vi "Fix_multi_header_bug.vi"(1 "Raw data File to Read":path) -> (0 "Raw data File to Read Out":path)   [LabVIEW 2010]
uses:
  Globals/Meas_global.vi
  Globals/Constants_global.vi
panel:
  out "character string":string
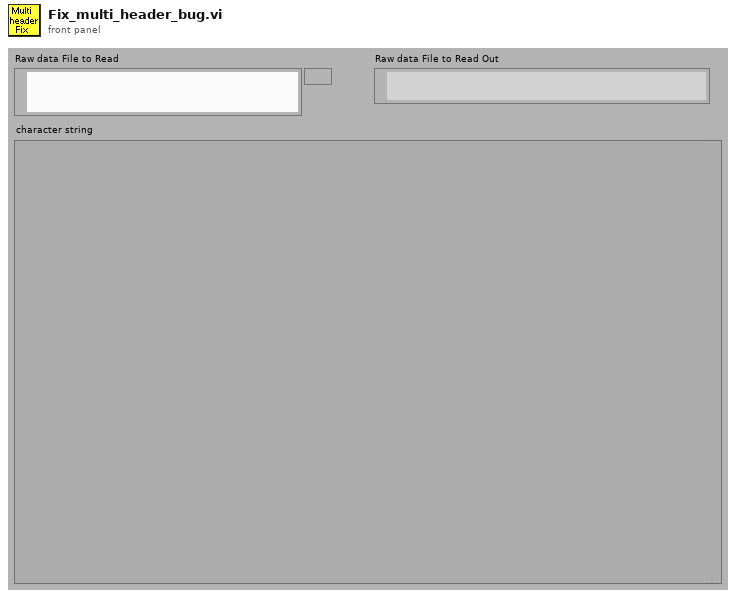
[diagram p1: front panel]
types:
  T1 = enum16{"read/write", "read-only", "write-only", "write-only (truncate)"}
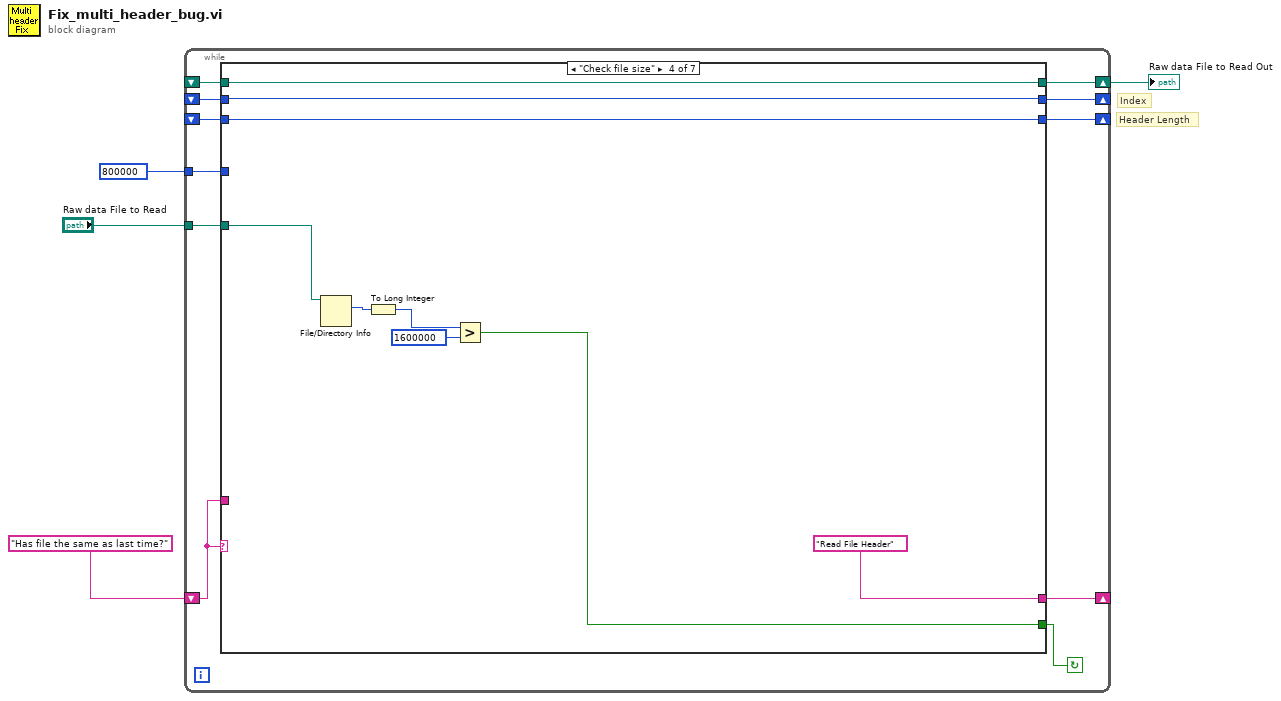
[diagram p0: block diagram]
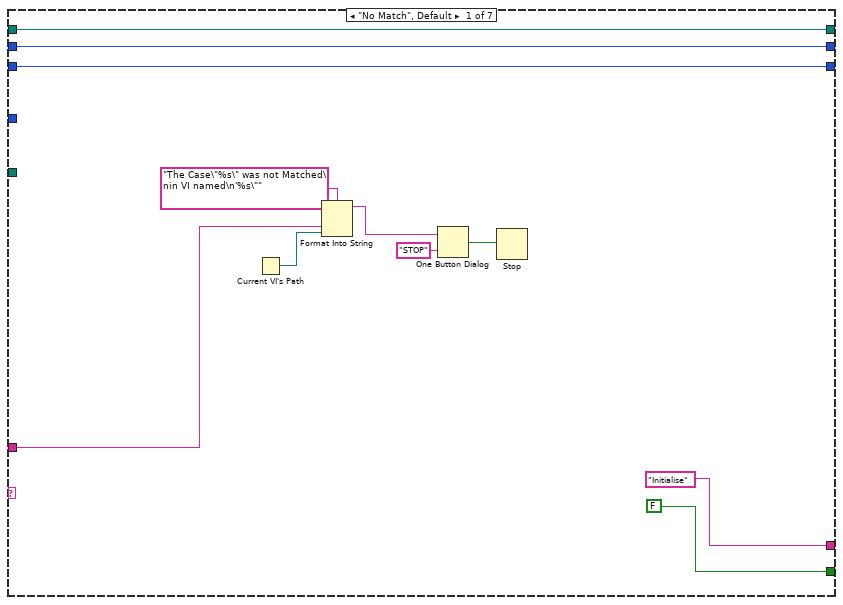
[diagram p2: hidden frame]
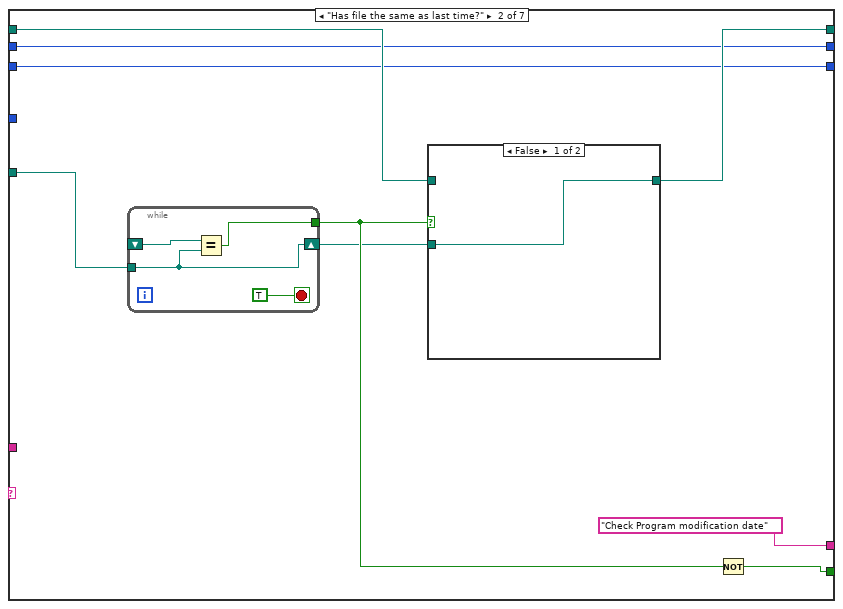
[diagram p3: hidden frame]
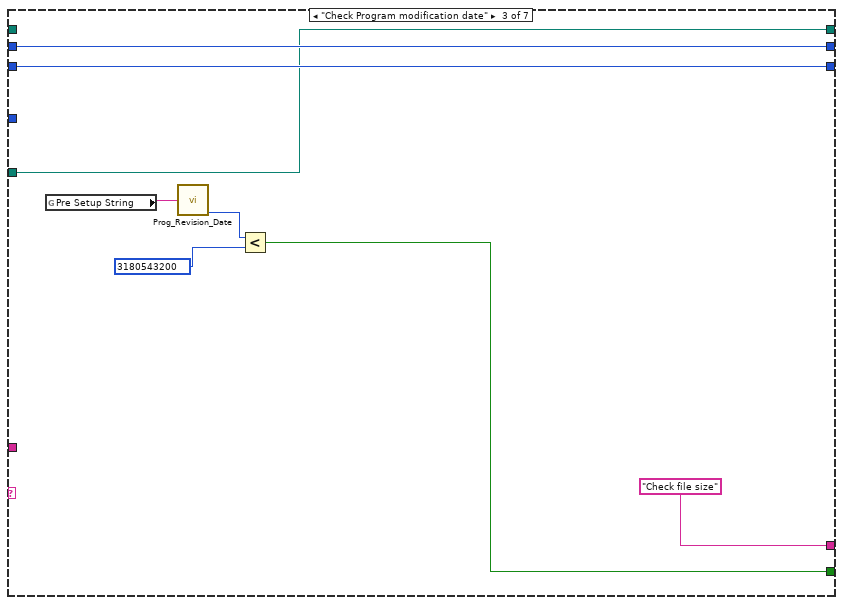
[diagram p5: hidden frame]
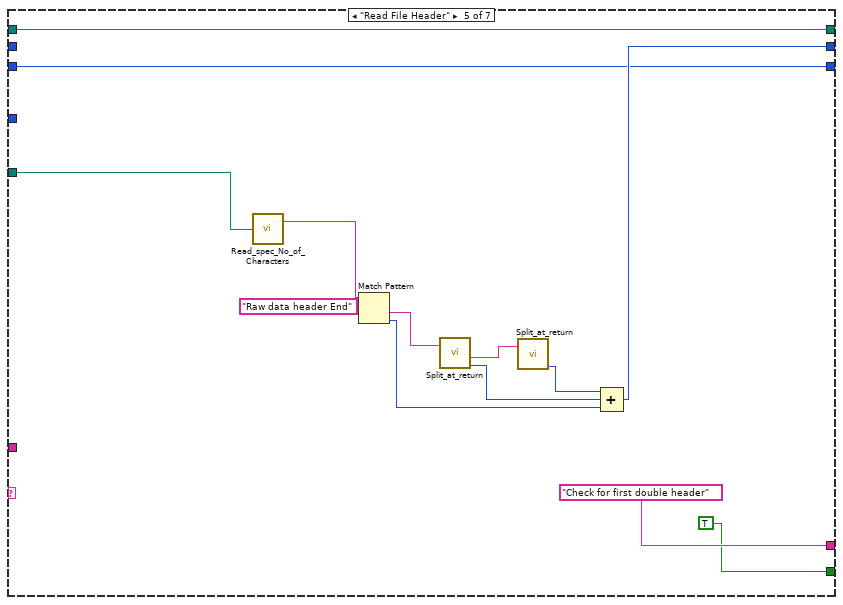
[diagram p6: hidden frame]
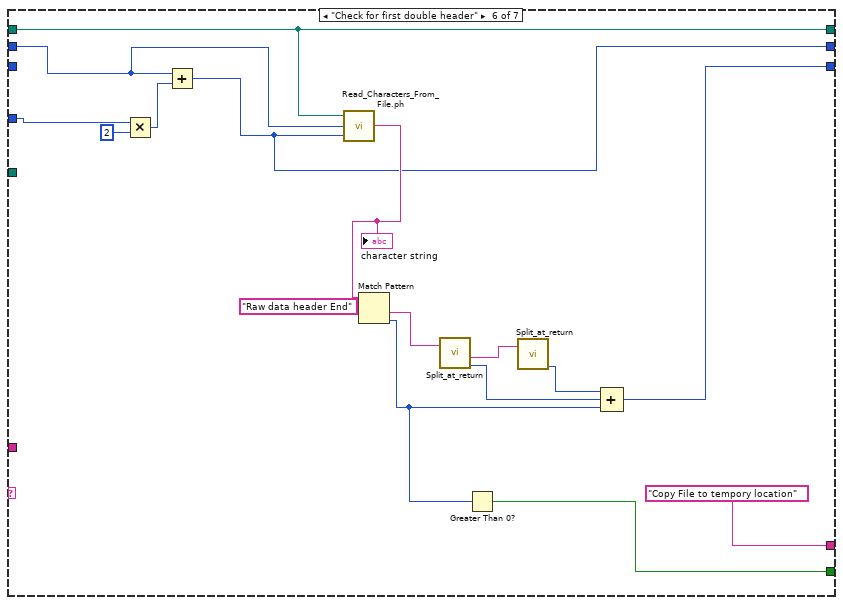
[diagram p7: hidden frame]
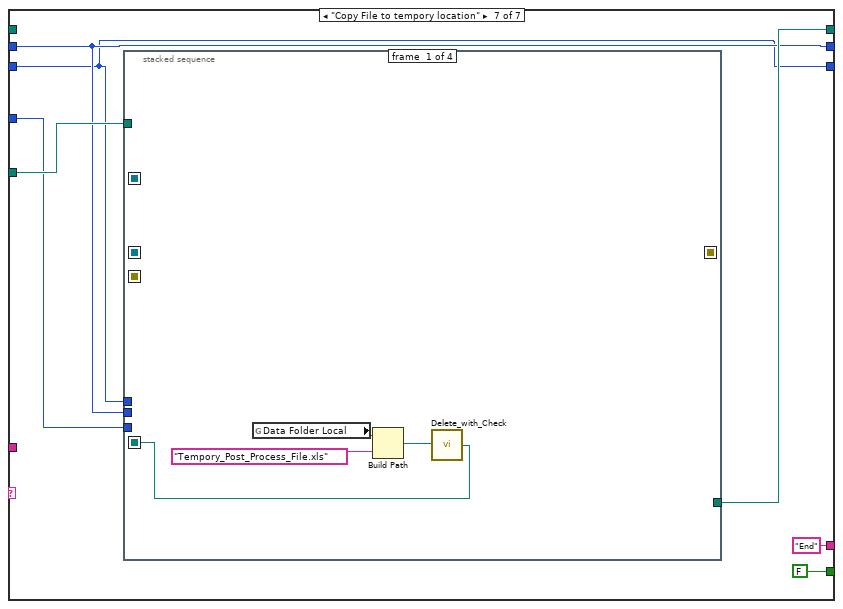
[diagram p8: hidden frame]
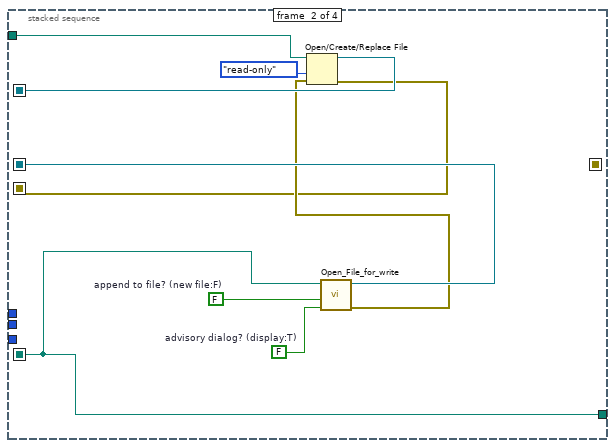
[diagram p9: hidden frame]
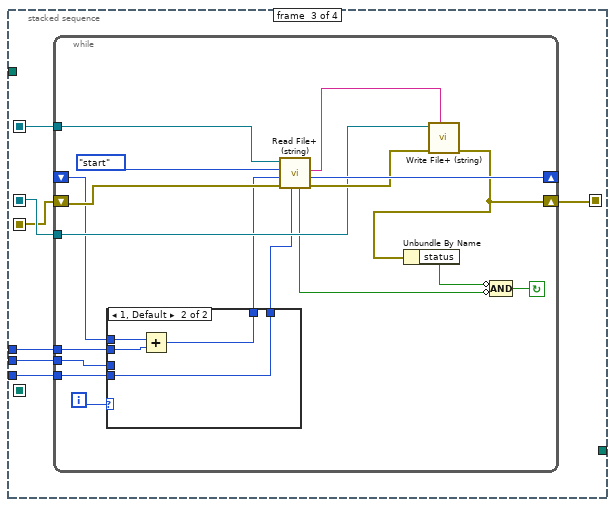
[diagram p10: hidden frame]
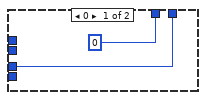
[diagram p11: hidden frame]
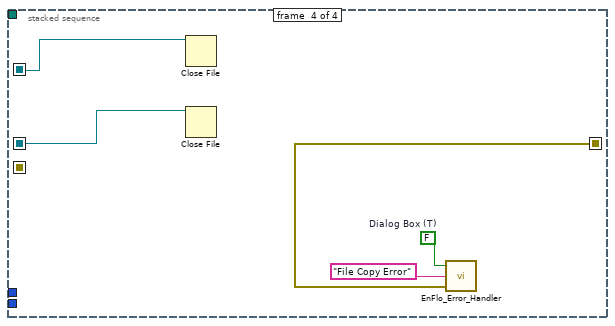
[diagram p12: hidden frame]
diagram:
  # "Header Length"
  # "Index"
  n1 = while {
    shift-left: "Has file the same as last time?" -> [w13]
    shift-right: [w14] -> _
    tunnel: "Raw data File to Read" -> [w12]
    shift-right: [w5] -> w2
    shift-left: _ -> [w11]
    shift-right: [w10] -> _
    shift-left: _ -> [w9]
    tunnel: 800000 -> [w8]
    shift-right: [w7] -> _
    shift-left: _ -> [w6]
    stop <- w15 continue-if-true
    n2 = case shown="\"Check file size\"" w13 {
      tunnel: [FALSE w29 w48 w54 TRUE w74 FALSE] -> w15
      tunnel: ["Initialise" "Check Program modification date" "Check file size" "Read File Header" "Check for first double header" "Copy File to tempory location" "End"] -> w14
      tunnel: w13 -> [w21 _ _ _ _ _ _]
      tunnel: w12 -> [_ w35 w44 w57 w69 _ w94]
      tunnel: [w18 w34 w44 w51 w68 w78 w93] -> w5
      tunnel: w11 -> [w18 w33 _ w51 w68 w78 _]
      tunnel: [w17 w32 w46 w53 w60 w72 w89] -> w10
      tunnel: w9 -> [w17 w32 w46 w53 _ w76 w89]
      tunnel: w8 -> [_ _ _ _ _ w81 w92]
      tunnel: [w16 w31 w45 w52 w59 w73 w88] -> w7
      tunnel: w6 -> [w16 w31 w45 w52 w59 _ w88]
      frame "No Match", Default {
        n3 = Current VI's Path() -> (path=w20:path)
        n4 = Format Into String(format string="The Case\"%s\" was not Matched\nin VI named\n'%s\"" ("Format String"), w21, w20) -> (resulting string=w24:string)  [unwired: 2 in, 1 out]
        n5 = One Button Dialog(message=w24, button name ("OK")="STOP") -> (true=w22:bool)
        n6 = Stop(stop? (T)=w22) -> ()
      }
      frame "Has file the same as last time?" {
        n7 = while {
          shift-right: [w41] -> w27
          shift-left: _ -> [w40]
          tunnel: w35 -> [w41]
          tunnel: [w39] -> w30
          stop <- TRUE stop-if-true
          n8 = Equal?(x=w40, y=w41) -> (x = y?=w39:bool)
        }
        n9 = case shown="False" w30 {
          tunnel: [w36 w37] -> w34
          tunnel: w33 -> [_ w37]
          tunnel: w27 -> [w36 _]
          frame False {
          }
          frame True {
          }
        }
        n10 = Not(x=w30) -> (.not. x?=w29:bool)
      }
      frame "Check Program modification date" {
        n11 = global read "Meas_global.vi" "Pre Setup String"() -> (w43:string)
        n12 = call "Prog_Revision_Date.vi"("Input string"=w43) -> ("Revision time (s)"=w42:u32)  [unwired: 4 out]
        n13 = Less?(x=w42, y=u32 3180543200 ("Prog's last revision date")) -> (x < y?=w48:bool)
      }
      frame "Check file size" {
        n14 = File/Directory Info(path=w57) -> (size=w50:i64)  [unwired: 1 in, 6 out]
        n15 = To Long Integer(number=w50) -> (32bit integer=w56:i32)
        n16 = Greater?(x=w56, y=1600000) -> (0:w54:bool)
      }
      frame "Read File Header" {
        n17 = call "Read_spec_No_of_Characters.vi"("Filename"=w69) -> ("character string"=w66:string)  [unwired: 1 out]
        n18 = Match Pattern(string=w66, regular expression="Raw data header End") -> (after substring=w64:string, offset past match=w62:i32)  [unwired: 3 out]
        n19 = call "Split_at_return.vi"("String"=w64) -> ("after substring"=w65:string, "offset past match"=w61:i32)  [unwired: 1 in, 2 out]
        n20 = call "Split_at_return.vi"("String"=w65) -> ("offset past match"=w63:i32)  [unwired: 1 in, 3 out]
        n21 = Compound Arithmetic op=ADD(w63, w61, w62) -> (w60:i32)
      }
      frame "Check for first double header" {
        n22 = Multiply(x=w81, y=2) -> (x*y=w80:i32)
        n23 = Add(x=w76, y=w80) -> (x+y=w72:i32)
        n24 = call "Read_Characters_From_File.ph.vi"("file path (dialog if empty)"=w78, "number of characters (all:-1)"=w76, "start of read offset (chars.: 0)"=w72) -> ("character string"=w77:string)  [unwired: 6 out]
        "character string" <- w77
        n25 = Match Pattern(string=w77, regular expression="Raw data header End") -> (after substring=w84:string, offset past match=w75:i32)  [unwired: 3 out]
        n26 = call "Split_at_return.vi"("String"=w84) -> ("after substring"=w85:string, "offset past match"=w82:i32)  [unwired: 1 in, 2 out]
        n27 = Greater Than 0?(x=w75) -> (x > 0?=w74:bool)
        n28 = call "Split_at_return.vi"("String"=w85) -> ("offset past match"=w83:i32)  [unwired: 1 in, 3 out]
        n29 = Compound Arithmetic op=ADD(w83, w82, w75) -> (w73:i32)
      }
      frame "Copy File to tempory location" {
        n30 = stacked-sequence {
          seq-local: [_ w104 _ _] -> [_ _ w114 w143]
          seq-local: [_ w106 _ _] -> [_ _ w113 w142]
          seq-local: [_ w102 _ _] -> [_ _ w112 _]
          seq-local: [_ _ w111 _] -> [_ _ _ w140]
          seq-local: [w95 _ _ _] -> [_ w99 _ _]
          tunnel: w94 -> [_ w100 _ _]
          tunnel: [_ w99 _ _] -> w93
          tunnel: w89 -> [_ _ w110 _]
          tunnel: w88 -> [_ _ w109 _]
          tunnel: w92 -> [_ _ w108 _]
          frame #0 {
            n31 = global read "Constants_global.vi" "Data Folder Local"() -> (w97:path)
            n32 = Build Path(base path=w97, name or relative path="Tempory_Post_Process_File.xls") -> (appended path=w96:path)
            n33 = call "Delete_with_Check.vi"("FilePath"=w96) -> ("Deleted Filepath"=w95:path)
          }
          frame #1 {
            w101 = FALSE  # advisory dialog? (display:T)
            w107 = FALSE  # append to file? (new file:F)
            n34 = call "Open_File_for_write.vi"("advisory dialog? (display:T)"=w101, "append to file? (new file:F)"=w107, "file path"=w99) -> ("error out"=w103:errorcluster, "refnum"=w106:refnum<file>)  [unwired: 7 out]
            n35 = Open/Create/Replace File(file path (use dialog)=w100, error in=w103, access (0:read/write)=T1."read-only" ("open mode (0)")) -> (refnum out=w104:refnum<file>, error out=w102:errorcluster)  [unwired: 4 out]
          }
          frame #2 {
            n36 = while {
              shift-left: w112 -> [w126]
              shift-right: [w125] -> w111
              tunnel: w113 -> [w128]
              shift-left: _ -> [w117]
              shift-right: [w130] -> _
              tunnel: w114 -> [w131]
              tunnel: w110 -> [w119]
              tunnel: w109 -> [w116]
              tunnel: w108 -> [w115]
              i -> [w121]
              stop <- w122 continue-if-true
              n37 = case shown="1, Default" w121 {
                tunnel: [w134 w135] -> w120
                tunnel: w119 -> [w134 _]
                tunnel: [0 ("mark after read (bytes)") w136] -> w118
                tunnel: w117 -> [_ w138]
                tunnel: w116 -> [_ w137]
                tunnel: w115 -> [_ w135]
                frame 0 {
                }
                frame 1, Default {
                  n38 = Add(x=w138, y=w137) -> (x+y=w136:i32)
                }
              }
              n39 = call <vilib>:"Read File+ (string).vi"("count"=w120, "error in (no error)"=w126, "pos offset (bytes:0)"=w118, "pos mode (rel. to current:2)"=enum16{"start", "end", "current"}."start", "refnum"=w131) -> ("error out"=w129:errorcluster, "mark after read (bytes)"=w130:i32, "string"=w127:string, "EOF?"=w123:bool)  [unwired: 3 out]
              n40 = call <vilib>:"Write File+ (string).vi"("string"=w127, "error in (no error)"=w129, "refnum"=w128) -> ("error out"=w125:errorcluster)  [unwired: 2 in, 4 out]
              n41 = Unbundle By Name(w125) -> ("status"=w124:bool)
              n42 = Compound Arithmetic op=AND(invert w124, invert w123) -> (w122:bool)
            }
          }
          frame #3 {
            w141 = FALSE  # Dialog Box (T)
            n43 = Close File(refnum=w143) -> ()  [unwired: 1 in, 2 out]
            n44 = Close File(refnum=w142) -> ()  [unwired: 1 in, 2 out]
            n45 = call "EnFlo_Error_Handler.vi"("error in (no error)"=w140, "Error Type"="File Copy Error", "Dialog Box (T)"=w141) -> ()  [unwired: 3 out]
          }
        }
      }
    }
  }
  "Raw data File to Read Out" <- w2
